vi "Initialise Inside Process (Base).vi"(8 "error in (no error)":errorcluster, 10 "Process":refnum<vi>, 11 "Actor in":refnum<class "Actor.lvclass">) -> (0 "error out":errorcluster, 3 "Actor out":refnum<class "Actor.lvclass">, 5 "Mailbox":refnum<event-registration>)   [LabVIEW 2020, in "Actor.lvclass"]
uses:
  Actor.lvclass
  Message.ctl
  Actor.lvclass/Actor.ctl
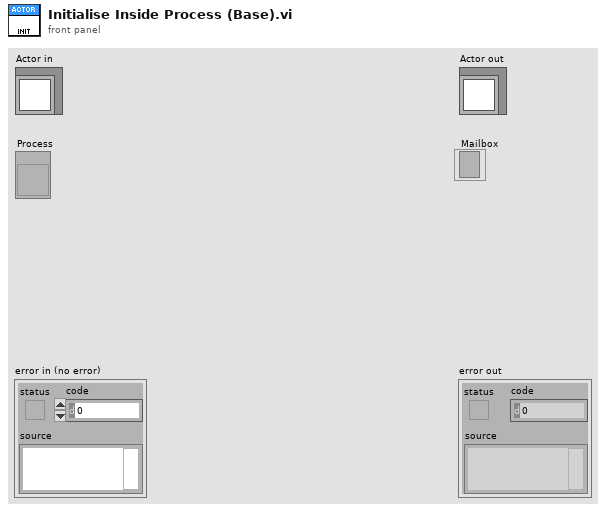
[diagram p1: front panel]
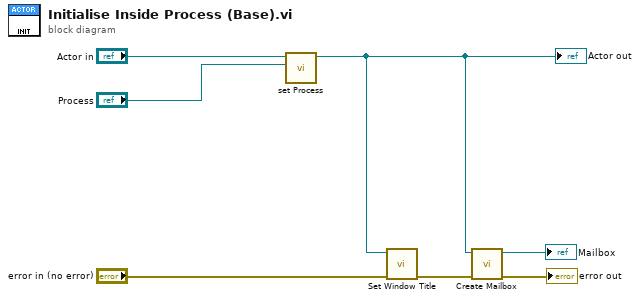
[diagram p0: block diagram]
diagram:
  n1 = call "set Process.vi"("Process"="Process", "Actor in"="Actor in") -> ("Actor out"=w3:refnum<class "Actor.lvclass">)  [unwired: 9 in]
  "Actor out" <- w3
  n2 = call "Set Window Title.vi"("error in (no error)"="error in (no error)", "Actor in"=w3) -> ("error out"=w5:errorcluster)  [unwired: 9 in]
  n3 = call "Create Mailbox.vi"("error in (no error)"=w5, "Actor in"=w3) -> ("error out"=→"error out":errorcluster, "Mailbox"=→"Mailbox":refnum<event-registration>)  [unwired: 8 in]
